vi "SSL UDP Receiver.vi"(10 "SSL Vision Address:":string="224.5.23.2", 11 "Port:":u16=10020) -> (0 "error out":errorcluster, 2 "Boolean":bool, 3 "Channel out":T1)   [LabVIEW 2016]
uses:
  <extravilib>/ChannelInstances/Lossy Stream-a[.](u8)/)Channel.ctl
  <extravilib>/ChannelInstances/Lossy Stream-a[.](u8)/Write With Abort.vi
  <extravilib>/ChannelInstances/Lossy Stream-a[.](u8)/Endpoint.vi
  <extravilib>/ChannelInstances/Lossy Stream-a[.](u8)/)Channel.vi
  <resource>/ChannelSupport/_ChannelSupport/WaitIfNeeded.vi
  <vilib>/Utility/tcp.llb/UDP Multicast Read-Only Open.vi
  <extravilib>/ChannelInstances/Lossy Stream-a[.](u8).lvlib
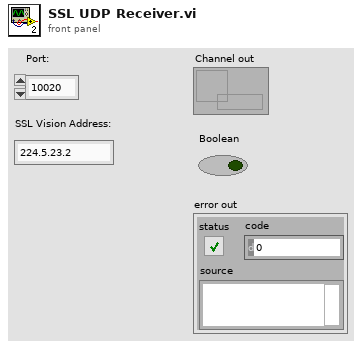
[diagram p1: front panel]
types:
  T1 = typedef "Lossy Stream-a[.](u8).lvlib/)Channel.ctl" = refnum<queue>
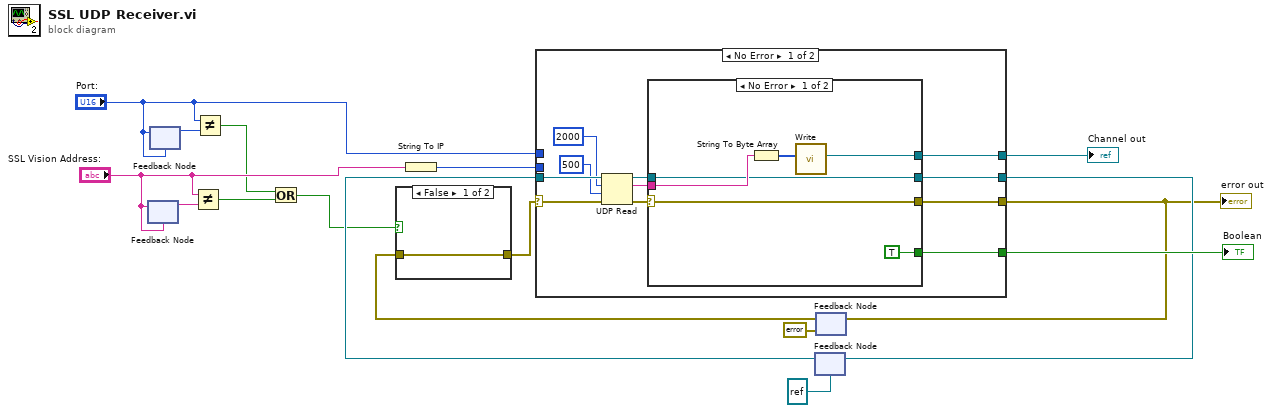
[diagram p0: block diagram]
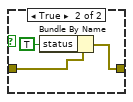
[diagram p2: hidden frame]
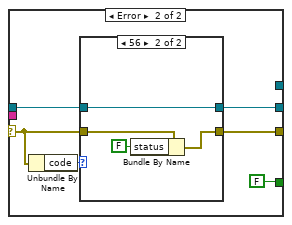
[diagram p3: hidden frame]
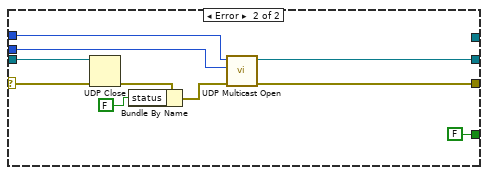
[diagram p5: hidden frame]
diagram:
  n1 = feedback-in #1("SSL Vision Address:") -> ()
  n2 = feedback #1("SSL Vision Address:") -> (w7:string)
  n3 = feedback #2("Port:") -> (w4:u16)
  n4 = feedback-in #2("Port:") -> ()
  n5 = Not Equal?(x="SSL Vision Address:", y=w7) -> (x != y?=w5:bool)
  n6 = Not Equal?(x="Port:", y=w4) -> (x != y?=w2:bool)
  n7 = Or(x=w2, y=w5) -> (x .or. y?=w1:bool)
  n8 = String To IP(1:"SSL Vision Address:") -> (0:w12:u32)
  n9 = feedback #3(refnum<k16> refnum ("connection ID")) -> (w14:refnum<k16>)
  n10 = feedback #4(errorcluster {"status"=TRUE, "code"=0, "source"=""} ("error out")) -> (w9:errorcluster)
  n11 = case shown="False" w1 {
    tunnel: w9 -> [w18 w20]
    tunnel: [w18 w19] -> w8
    frame False {
    }
    frame True {
      n12 = Bundle By Name(cluster=w20, "status"=TRUE) -> (w19:errorcluster)
    }
  }
  n13 = case shown="No Error" w8 {
    selector: w8 -> [w22 w51]
    tunnel: w14 -> [w32 w57]
    tunnel: [w31 _] -> w16
    tunnel: [w30 w59] -> w13
    tunnel: [w29 w60] -> w15
    tunnel: "Port:" -> [_ w58]
    tunnel: w12 -> [_ w56]
    tunnel: [w23 FALSE] -> w17
    frame No Error {
      n14 = UDP Read(connection ID=w32, max size (548)=2000, timeout ms (25000)=500, 8:w22) -> (data out=w26:string, error out=w24:errorcluster, 3:w25:refnum<k16>)  [unwired: 2 out]
      n15 = case shown="No Error" w24 {
        selector: w24 -> [w33 w39]
        tunnel: [w35 _] -> w31
        tunnel: w26 -> [w38 _]
        tunnel: [w33 w41] -> w30
        tunnel: [w37 w42] -> w29
        tunnel: w25 -> [w37 w43]
        tunnel: [TRUE FALSE] -> w23
        frame No Error {
          n16 = String To Byte Array(string=w38) -> (unsigned byte array=w36:u8[])
          n17 = call <extravilib>:"Write.vi"("element"=w36) -> ("channel"=w35:T1)  [unwired: 8 in, 2 out]
        }
        frame Error {
          n18 = Unbundle By Name(w39) -> ("code"=w44:i32)
          n19 = case shown="56" w44 {
            tunnel: w39 -> [w46 w50]
            tunnel: [w46 w48] -> w41
            tunnel: w43 -> [w45 w47]
            tunnel: [w45 w47] -> w42
            frame Default {
            }
            frame 56 {
              n20 = Bundle By Name(cluster=w50, "status"=FALSE) -> (w48:errorcluster)
            }
          }
        }
      }
    }
    frame Error {
      n21 = UDP Close(connection ID=w57, 8:w51) -> (error out=w54:errorcluster)  [unwired: 1 out]
      n22 = Bundle By Name(cluster=w54, "status"=FALSE) -> (w52:errorcluster)
      n23 = call-poly <vilib>:"UDP Multicast Open.vi"("error in (no error)"=w52, "multicast addr"=w56, "port"=w58) -> ("error out"=w59:errorcluster, "connection ID"=w60:refnum<k16>)  [unwired: 6 in, 1 out]
    }
  }
  "Boolean" <- w17
  "error out" <- w13
  "Channel out" <- w16
  n24 = feedback-in #3(w15) -> ()
  n25 = feedback-in #4(w13) -> ()
